vi "test_draw_pixmap.vi"() -> ()   [LabVIEW 2019]
panel:
  out "pict":picture
  in  "display_2":bool
  in  "display_1":bool
  in  "stop":bool
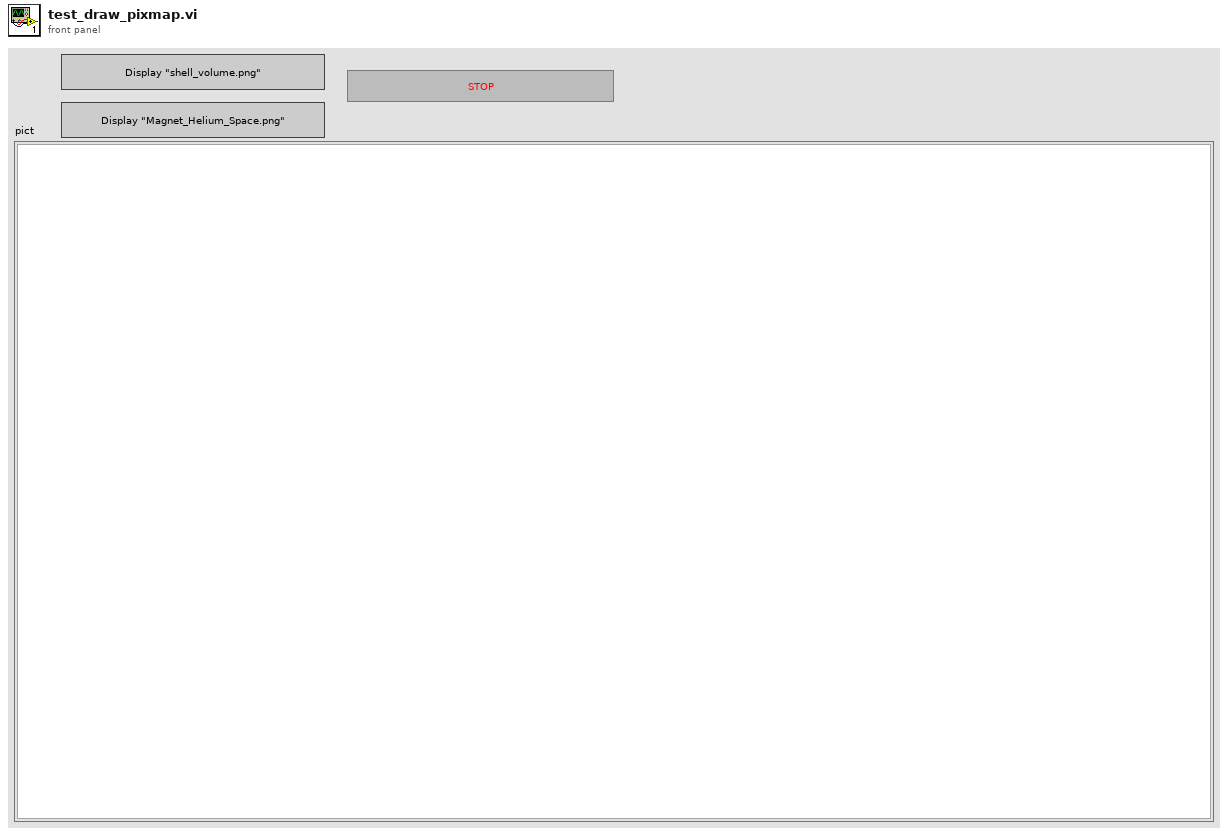
[diagram p1: front panel]
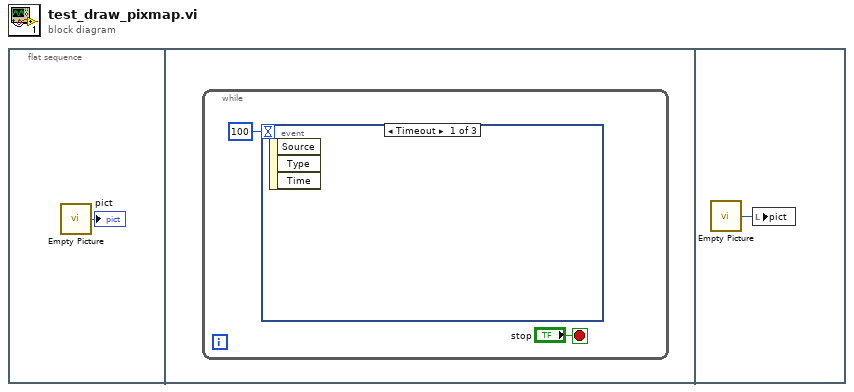
[diagram p0: block diagram]
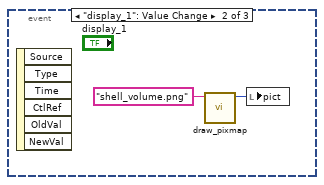
[diagram p2: hidden frame]
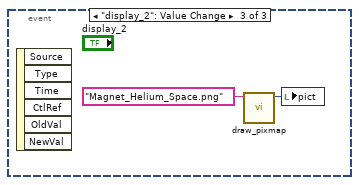
[diagram p3: hidden frame]
diagram:
  n1 = flat-sequence {
    frame #0 {
      n2 = call "Empty Picture"() -> ("empty picture"=→"pict":picture)
    }
    frame #1 {
      n3 = while {
        stop <- "stop" stop-if-true
        n4 = event shown="[0] Timeout" {
          selector: _ -> [_ _ _]
          dyn-events: _ -> [_ _ _]
          timeout: 100 -> [_ _ _]
          event Timeout {
            n5 = event-data() -> ()  [unwired: 1 in, 3 out]
          }
          event "display_1": Value Change {
            n6 = event-data() -> ()  [unwired: 1 in, 6 out]
            n7 = call "draw_pixmap.vi"("file_name"="shell_volume.png") -> ("pict"=w4:picture)  [unwired: 7 in, 3 out]
            n8 = local write "pict"(w4) -> ()
          }
          event "display_2": Value Change {
            n9 = event-data() -> ()  [unwired: 1 in, 6 out]
            n10 = call "draw_pixmap.vi"("file_name"="Magnet_Helium_Space.png") -> ("pict"=w6:picture)  [unwired: 7 in, 3 out]
            n11 = local write "pict"(w6) -> ()
          }
        }
      }
    }
    frame #2 {
      n12 = call "Empty Picture"() -> ("empty picture"=w8:picture)
      n13 = local write "pict"(w8) -> ()
    }
  }
